vi "svx_DAQ_UpdatePanel.vi"(2 "XControl Ref":refnum<vi>, 5 "State":T2={"Channel Info Array"=[], "Timing Mode"=enum."Time", "Timing Control 1"=25600.0, "Timing Control 2"=2560.0, "Timing Control 3"=16, "Timing Indicator 1"=0.1, "Reference Visible?"=FALSE, "Reference Type"=enum."<none>", "Tachometer Channel"="", "Tach Pulses Per Rev"=1, "Tach Direction"=enum."CW", "Tach Slope"=enum."Rising", "Tach Threshold"=0.0, "Trigger Channel"="", "Trigger Level"=20.0, "Pretrigger Samples"=1, "Trigger Slope"=enum."Falling", "Trigger Hysteresis"=0.0, "Logging Visible?"=FALSE, "Enable Logging"=FALSE, "Logfile Path"=path "c:/test.tdms"} {"Timing Control 2" format="%#_6f"; "Channel Info Array"."Max" min=0.0 format="± %^#_4g"; "Channel Info Array"."Channel Type" items=["Voltage (V)"=0, "Charge (C)"=9, "-"=99, "SPL (Pa)"=3, "Force (lbf)"=6, "Force (N)"=1, "Acceleration (g) - IEPE"=2, "Acceleration (g) - Charge"=12, "Acceleration (g) - 4 wire DC Voltage"=22, "Velocity (in/s)"=7, "Velocity (mm/s)"=8, "Prox Probe (mil)"=4, "Prox Probe (mm)"=5]}, 9 "cluster":T1, 11 "error in (no error)":errorcluster, 12 "display state change":bool) -> (6 "State Out":T2={"Channel Info Array"=[], "Timing Mode"=enum."Time", "Timing Control 1"=25600.0, "Timing Control 2"=2560.0, "Timing Control 3"=16, "Timing Indicator 1"=0.1, "Reference Visible?"=FALSE, "Reference Type"=enum."<none>", "Tachometer Channel"="", "Tach Pulses Per Rev"=1, "Tach Direction"=enum."CW", "Tach Slope"=enum."Rising", "Tach Threshold"=0.0, "Trigger Channel"="", "Trigger Level"=20.0, "Pretrigger Samples"=1, "Trigger Slope"=enum."Falling", "Trigger Hysteresis"=0.0, "Logging Visible?"=FALSE, "Enable Logging"=FALSE, "Logfile Path"=path "c:/test.tdms"} caption="State" {"Timing Control 2" format="%#_6f"; "Channel Info Array"."Max" min=0.0 format="± %^#_4g"; "Channel Info Array"."Channel Type" items=["Voltage (V)"=0, "Charge (C)"=9, "-"=99, "SPL (Pa)"=3, "Force (lbf)"=6, "Force (N)"=1, "Acceleration (g) - IEPE"=2, "Acceleration (g) - Charge"=12, "Acceleration (g) - 4 wire DC Voltage"=22, "Velocity (in/s)"=7, "Velocity (mm/s)"=8, "Prox Probe (mil)"=4, "Prox Probe (mm)"=5]}, 10 "cluster":T1, 15 "error out":errorcluster)   [LabVIEW 2017, in "SVX NI-DAQmx AI Configuration XControl.xctl"]
uses:
  <vilib>/addons/Sound and Vibration/svt_DAQmx/Configuration XControl/SVX NI-DAQmx AI Configuration XControl.xctl
  <vilib>/addons/Sound and Vibration/svt_DAQmx/Configuration XControl/SubVIs/svx_DAQ_State.ctl
  <vilib>/addons/Sound and Vibration/svt_DAQmx/Configuration XControl/Controls/svx_DAQ_ChannelInfo.ctl
  <vilib>/addons/Sound and Vibration/svt_DAQmx/Configuration XControl/Controls/svx_DAQ_ChannelType.ctl
  <vilib>/addons/Sound and Vibration/svt_DAQmx/Configuration XControl/Controls/svx_DAQ_Coupling.ctl
  <vilib>/addons/Sound and Vibration/svt_DAQmx/Configuration XControl/Controls/svx_DAQ_Excitation.ctl
  <vilib>/addons/Sound and Vibration/svt_DAQmx/Configuration XControl/Controls/svx_DAQ_TimingType.ctl
  <vilib>/addons/Sound and Vibration/svt_DAQmx/Configuration XControl/Controls/svx_DAQ_ReferenceType.ctl
  <vilib>/addons/Sound and Vibration/svt_DAQmx/Configuration XControl/Controls/svx_DAQ_RotationDirection.ctl
  <vilib>/addons/Sound and Vibration/svt_DAQmx/Configuration XControl/Controls/svx_DAQ_Tach_Slope.ctl
  <vilib>/addons/Sound and Vibration/svt_DAQmx/Configuration XControl/Controls/svx_DAQ_Trigger_Slope.ctl
  <vilib>/addons/Sound and Vibration/svt_DAQmx/Configuration XControl/Controls/svx_DAQ_ControlRefs.ctl
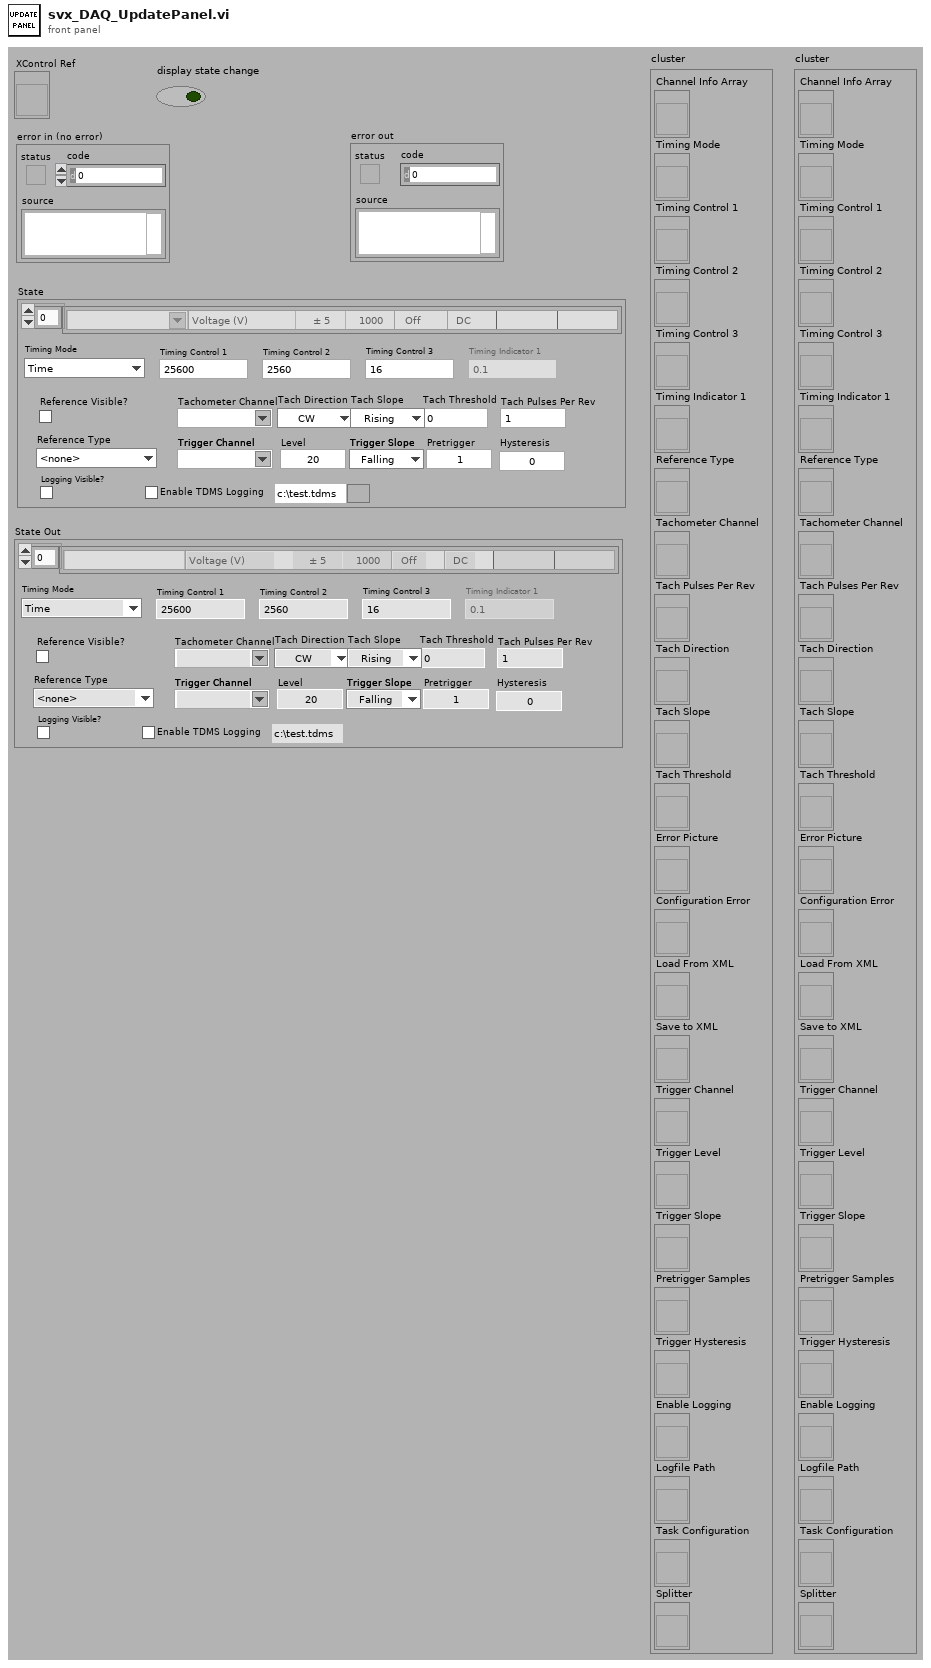
[diagram p1: front panel]
types:
  T1 = typedef "SVX NI-DAQmx AI Configuration XControl.xctl/svx_DAQ_ControlRefs.ctl" = cluster{"Channel Info Array":refnum<vi>, "Timing Mode":refnum<vi>, "Timing Control 1":refnum<vi>, "Timing Control 2":refnum<vi>, "Timing Control 3":refnum<vi>, "Timing Indicator 1":refnum<vi>, "Reference Type":refnum<vi>, "Tachometer Channel":refnum<vi>, "Tach Pulses Per Rev":refnum<vi>, "Tach Direction":refnum<vi>, "Tach Slope":refnum<vi>, "Tach Threshold":refnum<vi>, "Error Picture":refnum<vi>, "Configuration Error":refnum<vi>, "Load From XML":refnum<vi>, "Save to XML":refnum<vi>, "Trigger Channel":refnum<vi>, "Trigger Level":refnum<vi>, "Trigger Slope":refnum<vi>, "Pretrigger Samples":refnum<vi>, "Trigger Hysteresis":refnum<vi>, "Enable Logging":refnum<vi>, "Logfile Path":refnum<vi>, "Task Configuration":refnum<vi>, "Splitter":refnum<vi>}
  T2 = typedef "SVX NI-DAQmx AI Configuration XControl.xctl/svx_DAQ_State.ctl" = cluster{"Channel Info Array":T3[], "Timing Mode":T7, "Timing Control 1":dbl, "Timing Control 2":dbl, "Timing Control 3":i32, "Timing Indicator 1":dbl, "Reference Visible?":bool, "Reference Type":T8, "Tachometer Channel":string, "Tach Pulses Per Rev":i32, "Tach Direction":T9, "Tach Slope":T10, "Tach Threshold":dbl, "Trigger Channel":string, "Trigger Level":dbl, "Pretrigger Samples":i32, "Trigger Slope":T11, "Trigger Hysteresis":dbl, "Logging Visible?":bool, "Enable Logging":bool, "Logfile Path":path}
  T3 = typedef "SVX NI-DAQmx AI Configuration XControl.xctl/svx_DAQ_ChannelInfo.ctl" = cluster{"Initialized?":bool, "DAQmx Channel":tag, "Channel Type":T4, "Max":dbl, "Sensitivity":dbl, "Excitation":bool, "Coupling":T5, "Location":string, "Orientation":string, "excitation":T6}
  T4 = typedef "SVX NI-DAQmx AI Configuration XControl.xctl/svx_DAQ_ChannelType.ctl" = u16
  T5 = typedef "SVX NI-DAQmx AI Configuration XControl.xctl/svx_DAQ_Coupling.ctl" = enum16{"AC", "DC"}
  T6 = typedef "svx_DAQ_Excitation.ctl" = enum16{"Off", "Min", "Max"}
  T7 = typedef "SVX NI-DAQmx AI Configuration XControl.xctl/svx_DAQ_TimingType.ctl" = enum16{"Time", "Frequency", "Order"}
  T8 = typedef "SVX NI-DAQmx AI Configuration XControl.xctl/svx_DAQ_ReferenceType.ctl" = enum16{"<none>", "Analog Tachometer", "Analog SW Trigger"}
  T9 = typedef "SVX NI-DAQmx AI Configuration XControl.xctl/svx_DAQ_RotationDirection.ctl" = enum16{"CW", "CCW"}
  T10 = typedef "SVX NI-DAQmx AI Configuration XControl.xctl/svx_DAQ_Tach_Slope.ctl" = enum16{"Rising", "Falling"}
  T11 = typedef "SVX NI-DAQmx AI Configuration XControl.xctl/svx_DAQ_Trigger_Slope.ctl" = enum16{"Falling", "Rising"}
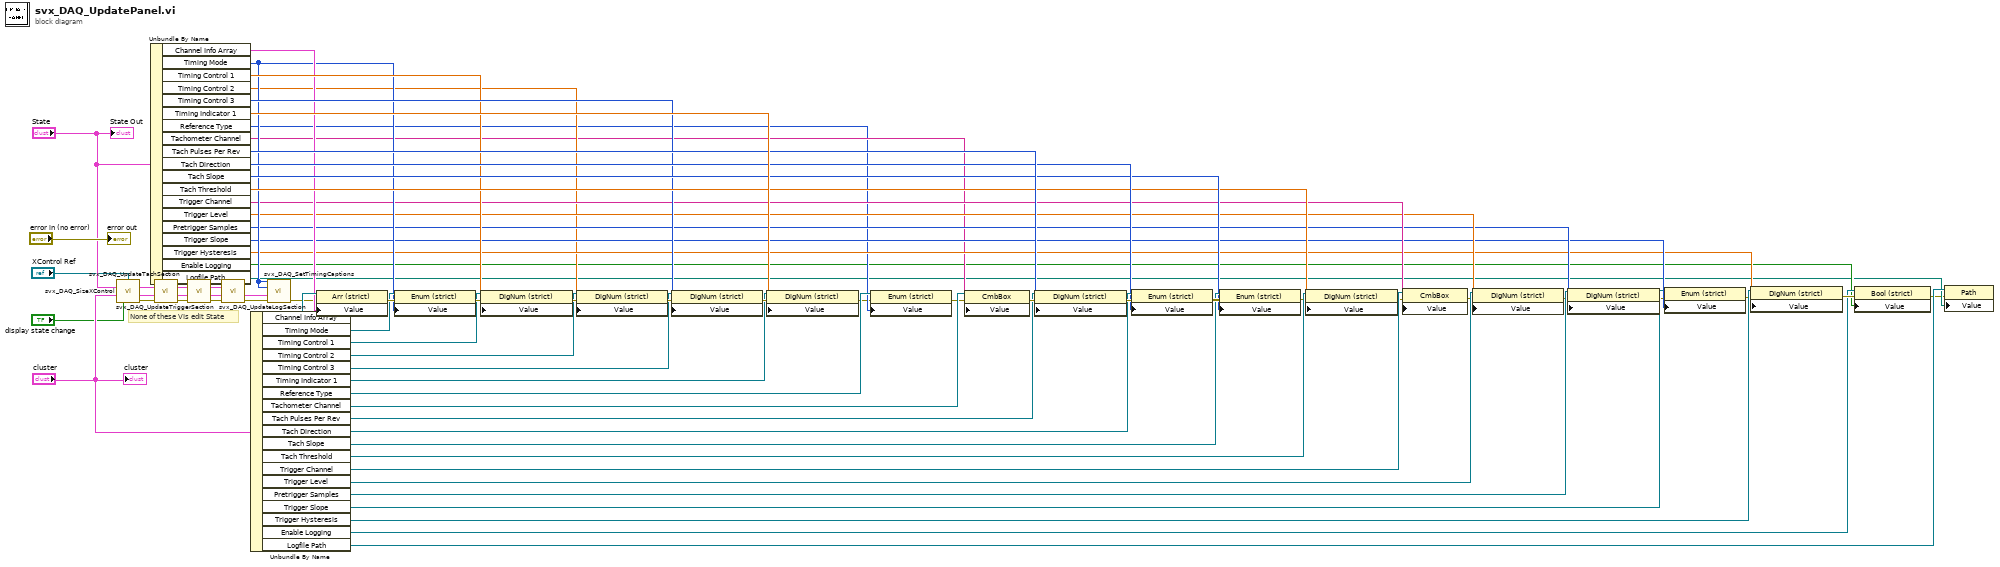
[diagram p0: block diagram]
diagram:
  # "None of these VIs edit State"
  n1 = call <vilib>:"svx_DAQ_SizeXControl.vi"("XControl Ref"="XControl Ref", "State"="State", "Reference Cluster"="cluster", "display state change"="display state change") -> ("State Out"=w6:T2, "Reference Cluster Out"=w7:T1, "error out"=w10:errorcluster)  [unwired: 9 in]
  n2 = Unbundle By Name("State") -> ("Channel Info Array"=w47:T3[], "Timing Mode"=w46:T7, "Timing Control 1"=w48:dbl, "Timing Control 2"=w25:dbl, "Timing Control 3"=w49:i32, "Timing Indicator 1"=w60:dbl, "Reference Type"=w21:T8, "Tachometer Channel"=w24:string, "Tach Pulses Per Rev"=w58:i32, "Tach Direction"=w56:T9, "Tach Slope"=w53:T10, "Tach Threshold"=w52:dbl, "Trigger Channel"=w39:string, "Trigger Level"=w38:dbl, "Pretrigger Samples"=w35:i32, "Trigger Slope"=w34:T11, "Trigger Hysteresis"=w31:dbl, "Enable Logging"=w16:bool, "Logfile Path"=w3:path)
  n3 = call <vilib>:"svx_DAQ_UpdateTachSection.vi"("State"=w6, "cluster"=w7, "error in (no error)"=w10) -> ("State Out"=w43:T2, "cluster"=w41:T1, "error out"=w42:errorcluster)  [unwired: 10 in]
  n4 = call <vilib>:"svx_DAQ_UpdateTriggerSection.vi"("State"=w43, "Reference Cluster"=w41, "error in (no error)"=w42) -> ("State Out"=w13:T2, "Reference Cluster Out"=w15:T1, "error out"=w14:errorcluster)  [unwired: 10 in]
  n5 = call <vilib>:"svx_DAQ_UpdateLogSection.vi"("State"=w13, "Reference Cluster"=w15, "error in (no error)"=w14) -> ("Reference Cluster Out"=w11:T1, "error out"=w12:errorcluster)  [unwired: 10 in, 1 out]
  n6 = Unbundle By Name("cluster") -> ("Channel Info Array"=w73:refnum<vi>, "Timing Mode"=w65:refnum<vi>, "Timing Control 1"=w64:refnum<vi>, "Timing Control 2"=w63:refnum<vi>, "Timing Control 3"=w62:refnum<vi>, "Timing Indicator 1"=w61:refnum<vi>, "Reference Type"=w22:refnum<vi>, "Tachometer Channel"=w23:refnum<vi>, "Tach Pulses Per Rev"=w59:refnum<vi>, "Tach Direction"=w57:refnum<vi>, "Tach Slope"=w55:refnum<vi>, "Tach Threshold"=w54:refnum<vi>, "Trigger Channel"=w40:refnum<vi>, "Trigger Level"=w37:refnum<vi>, "Pretrigger Samples"=w36:refnum<vi>, "Trigger Slope"=w33:refnum<vi>, "Trigger Hysteresis"=w32:refnum<vi>, "Enable Logging"=w17:refnum<vi>, "Logfile Path"=w4:refnum<vi>)
  n7 = call <vilib>:"svx_DAQ_SetTimingCaptions.vi"("Timing Mode (new)"=w46, "Timing Mode (old)"=w46, "Reference Cluster"=w11, "error in (no error)"=w12) -> ("error out"=w44:errorcluster)  [unwired: 7 in, 4 out]
  n8 = property class="Arr (strict)"(reference=w73, error in=w44, "Value"=w47) -> (error out=w72:errorcluster)  [unwired: 1 out]
  n9 = property class="Enum (strict)"(reference=w65, error in=w72, "Value"=w46) -> (error out=w71:errorcluster)  [unwired: 1 out]
  n10 = property class="DigNum (strict)"(reference=w64, error in=w71, "Value"=w48) -> (error out=w70:errorcluster)  [unwired: 1 out]
  n11 = property class="DigNum (strict)"(reference=w63, error in=w70, "Value"=w25) -> (error out=w69:errorcluster)  [unwired: 1 out]
  n12 = property class="DigNum (strict)"(reference=w62, error in=w69, "Value"=w49) -> (error out=w68:errorcluster)  [unwired: 1 out]
  n13 = property class="DigNum (strict)"(reference=w61, error in=w68, "Value"=w60) -> (error out=w20:errorcluster)  [unwired: 1 out]
  n14 = property class="Enum (strict)"(reference=w22, error in=w20, "Value"=w21) -> (error out=w19:errorcluster)  [unwired: 1 out]
  n15 = property class="CmbBox"(reference=w23, error in=w19, "Value"=w24) -> (error out=w67:errorcluster)  [unwired: 1 out]
  n16 = property class="DigNum (strict)"(reference=w59, error in=w67, "Value"=w58) -> (error out=w66:errorcluster)  [unwired: 1 out]
  n17 = property class="Enum (strict)"(reference=w57, error in=w66, "Value"=w56) -> (error out=w51:errorcluster)  [unwired: 1 out]
  n18 = property class="Enum (strict)"(reference=w55, error in=w51, "Value"=w53) -> (error out=w50:errorcluster)  [unwired: 1 out]
  n19 = property class="DigNum (strict)"(reference=w54, error in=w50, "Value"=w52) -> (error out=w30:errorcluster)  [unwired: 1 out]
  n20 = property class="CmbBox"(reference=w40, error in=w30, "Value"=w39) -> (error out=w29:errorcluster)  [unwired: 1 out]
  n21 = property class="DigNum (strict)"(reference=w37, error in=w29, "Value"=w38) -> (error out=w28:errorcluster)  [unwired: 1 out]
  n22 = property class="DigNum (strict)"(reference=w36, error in=w28, "Value"=w35) -> (error out=w27:errorcluster)  [unwired: 1 out]
  n23 = property class="Enum (strict)"(reference=w33, error in=w27, "Value"=w34) -> (error out=w26:errorcluster)  [unwired: 1 out]
  n24 = property class="DigNum (strict)"(reference=w32, error in=w26, "Value"=w31) -> (error out=w18:errorcluster)  [unwired: 1 out]
  n25 = property class="Bool (strict)"(reference=w17, error in=w18, "Value"=w16) -> (error out=w2:errorcluster)  [unwired: 1 out]
  n26 = property class="Path"(reference=w4, error in=w2, "Value"=w3) -> ()  [unwired: 2 out]
  "State Out" <- "State"
  "error out" <- "error in (no error)"
  "cluster" <- "cluster"
